vi "ShiftToMapCoord.vi"(9 "Y abs":dbl, 10 "X abs":dbl) -> (1 "Y map":dbl, 2 "X map":dbl)   [LabVIEW 2009, in "Main.lvlib"]
uses:
  Main.lvlib
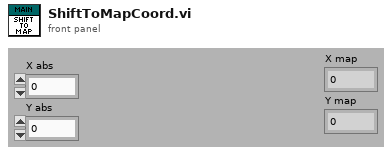
[diagram p1: front panel]
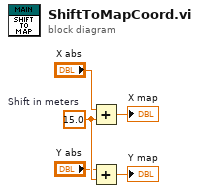
[diagram p0: block diagram]
diagram:
  w5 = 15.0  # Shift in meters
  n1 = Add(x="X abs", y=w5) -> (x+y=→"X map":dbl)
  n2 = Add(x="Y abs", y=w5) -> (x+y=→"Y map":dbl)
